vi "Start Asynchronus Logger.vi"(8 "error in (no error)":errorcluster, 10 "Queue in":refnum<queue>, 11 "Data Cluster OUT in":T1 {"Measurement Configuration"."Relative To" items=["Power sequence start", "Previous source start", "Previous source end"]; "Measurement Configuration"."Power line frequency" items=["50 Hz", "60 Hz"]; "Measurement Configuration"."Start Value" format="%#_6p"; "Measurement Configuration"."Transient Response" items=["Slow", "Normal", "Fast"]; "Measurement Configuration"."Sense Mode" items=["Local Sense", "Remote Sense"]; "Measurement Configuration"."Target Value" format="%#_6p"; "Measurement Configuration"."Source Mode" items=["DC Voltage", "DC Current"]; "Measurement Configuration"."Start Delay" format="%#_6p"; "Measurement Configuration"."Compliance Limit" format="%#_6p"; "Measurement Configuration"."Ramp Rate" format="%#_6p"}) -> (0 "error out":errorcluster, 3 "Data Cluster OUT out":T1 {"Measurement Configuration"."Relative To" items=["Power sequence start", "Previous source start", "Previous source end"]; "Measurement Configuration"."Power line frequency" items=["50 Hz", "60 Hz"]; "Measurement Configuration"."Start Value" format="%#_6p"; "Measurement Configuration"."Transient Response" items=["Slow", "Normal", "Fast"]; "Measurement Configuration"."Sense Mode" items=["Local Sense", "Remote Sense"]; "Measurement Configuration"."Target Value" format="%#_6p"; "Measurement Configuration"."Source Mode" items=["DC Voltage", "DC Current"]; "Measurement Configuration"."Start Delay" format="%#_6p"; "Measurement Configuration"."Compliance Limit" format="%#_6p"; "Measurement Configuration"."Ramp Rate" format="%#_6p"})   [LabVIEW 2024, in "devicePowerSequencerCoreLogic.lvlib"]
doc: "Starts the Asynchronous Logger to log measure data."
uses:
  devicePowerSequencerCoreLogic.lvlib
  controls/Data Cluster.ctl
  <vilib>/Plug-In SDKs/Clients/Session Management V1/Session Reservation/Session Reservation.lvclass
  <vilib>/Plug-In SDKs/Measurements/Measure Call Context/Measure Call Context.lvclass
  Measurement Configuration.ctl
  controls/Source Mode.ctl
  controls/Sense Mode.ctl
  controls/Relative To.ctl
  controls/Transient Response.ctl
  controls/Power line frequency.ctl
  Measurement Results.ctl
  controls/Channel Name.ctl
  controls/Software Flags.ctl
  controls/Ramp Configurations.ctl
  controls/Error Info.ctl
  controls/Measurements.ctl
  controls/Voltage and Current Measurements.ctl
  controls/Log Configurations.ctl
  Device Power Sequencer.lvlib
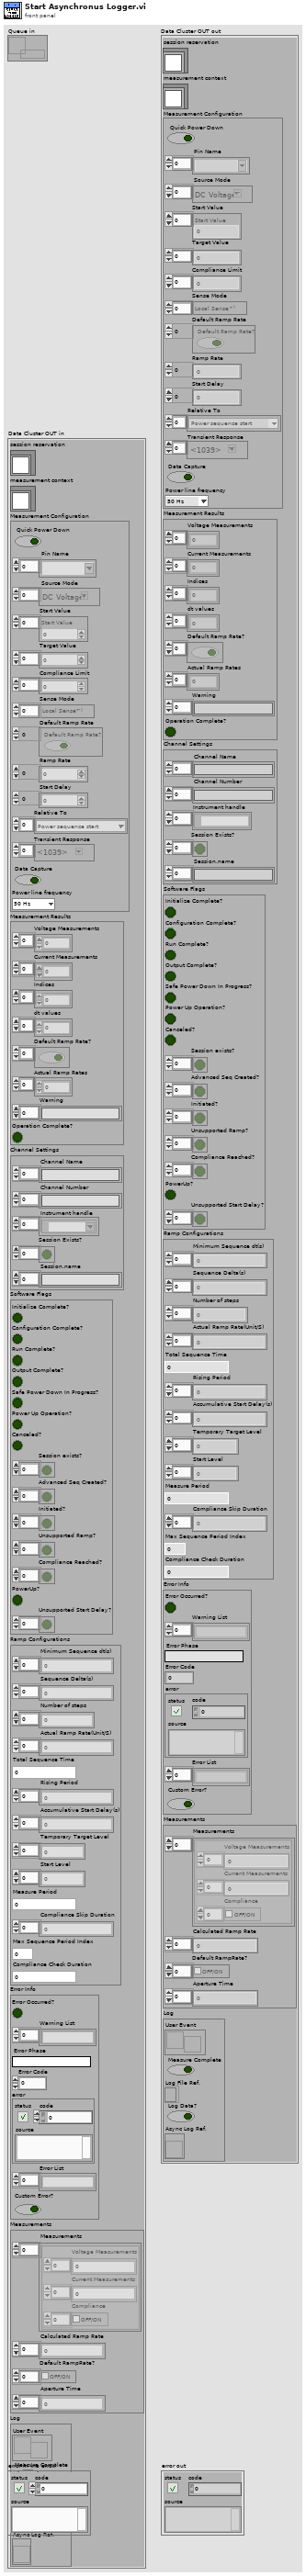
[diagram p1: front panel]
types:
  T1 = typedef "devicePowerSequencerCoreLogic.lvlib/Data Cluster.ctl" = cluster{"session reservation":refnum<class "Session Reservation.lvclass">, "measurement context":refnum<class "Measure Call Context.lvclass">, "Measurement Configuration":T2, "Measurement Results":T8, "Channel Settings":T9, "Software Flags":T10, "Ramp Configurations":T11, "Error Info":T12, "Measurements":T13, "Log":T15}
  T2 = typedef "Device Power Sequencer.lvlib/Measurement Configuration.ctl" = cluster{"Quick Power Down":bool, "Pin Name":string[], "Source Mode":T3[], "Start Value":dbl[], "Target Value":dbl[], "Compliance Limit":dbl[], "Sense Mode":T4[], "Default Ramp Rate":bool[], "Ramp Rate":dbl[], "Start Delay":dbl[], "Relative To":T5[], "Transient Response":T6[], "Data Capture":bool, "Power line frequency":T7}
  T3 = typedef "Device Power Sequencer.lvlib/Source Mode.ctl" = i32
  T4 = typedef "Device Power Sequencer.lvlib/Sense Mode.ctl" = i32
  T5 = typedef "Device Power Sequencer.lvlib/Relative To.ctl" = u32
  T6 = typedef "Device Power Sequencer.lvlib/Transient Response.ctl" = i32
  T7 = typedef "Device Power Sequencer.lvlib/Power line frequency.ctl" = u32
  T8 = typedef "Device Power Sequencer.lvlib/Measurement Results.ctl" = cluster{"Voltage Measurements":dbl[], "Current Measurements":dbl[], "Indices":i32[], "dt values":dbl[], "Default Ramp Rate?":bool[], "Actual Ramp Rates":dbl[], "Warning":string[], "Operation Complete?":bool}
  T9 = typedef "devicePowerSequencerCoreLogic.lvlib/Channel Name.ctl" = cluster{"Channel Name":string[], "Channel Number":string[], "Instrument handle":refnum<k15>[], "Session Exists?":bool[], "Session.name":string[]}
  T10 = typedef "devicePowerSequencerCoreLogic.lvlib/Software Flags.ctl" = cluster{"Initialize Complete?":bool, "Configuration Complete?":bool, "Run Complete?":bool, "Output Complete?":bool, "Safe Power Down In Progress?":bool, "Power Up Operation?":bool, "Canceled?":bool, "Session exists?":bool[], "Advanced Seq Created?":bool[], "Initiated?":bool[], "Unsupported Ramp?":bool[], "Compliance Reached?":bool[], "PowerUp?":bool, "Unsupported Start Delay?":bool[]}
  T11 = typedef "devicePowerSequencerCoreLogic.lvlib/Ramp Configurations.ctl" = cluster{"Minimum Sequence dt(s)":dbl[], "Sequence Delta(s)":dbl[], "Number of steps":i32[], "Actual Ramp Rate(Unit/S)":dbl[], "Total Sequence Time":dbl, "Rising Period":dbl[], "Accumulative Start Delay(s)":dbl[], "Temporary Target Level":dbl[], "Start Level":dbl[], "Measure Period":dbl, "Compliance Skip Duration":dbl[], "Max Sequence Period Index":i32, "Compliance Check Duration":dbl}
  T12 = typedef "devicePowerSequencerCoreLogic.lvlib/Error Info.ctl" = cluster{"Error Occurred?":bool, "Warning List":string[], "Error Phase":string, "Error Code":i32, "error":errorcluster, "Error List":string[], "Custom Error?":bool}
  T13 = typedef "devicePowerSequencerCoreLogic.lvlib/Measurements.ctl" = cluster{"Measurements":T14[], "Calculated Ramp Rate":dbl[], "Default RampRate?":bool[], "Aperture Time":dbl[]}
  T14 = typedef "devicePowerSequencerCoreLogic.lvlib/Voltage and Current Measurements.ctl" = cluster{"Voltage Measurements":dbl[], "Current Measurements":dbl[], "Compliance":bool[]}
  T15 = typedef "devicePowerSequencerCoreLogic.lvlib/Log Configurations.ctl" = cluster{"User Event":refnum<user-event>, "Measure Complete":bool, "Log File Ref.":refnum<file>, "Log Data?":bool, "Async Log Ref.":refnum<vi>}
  T16 = cluster{"Measured Data":cluster{"Voltage":dbl[], "Current":dbl[]}[], "Measure Complete":bool}
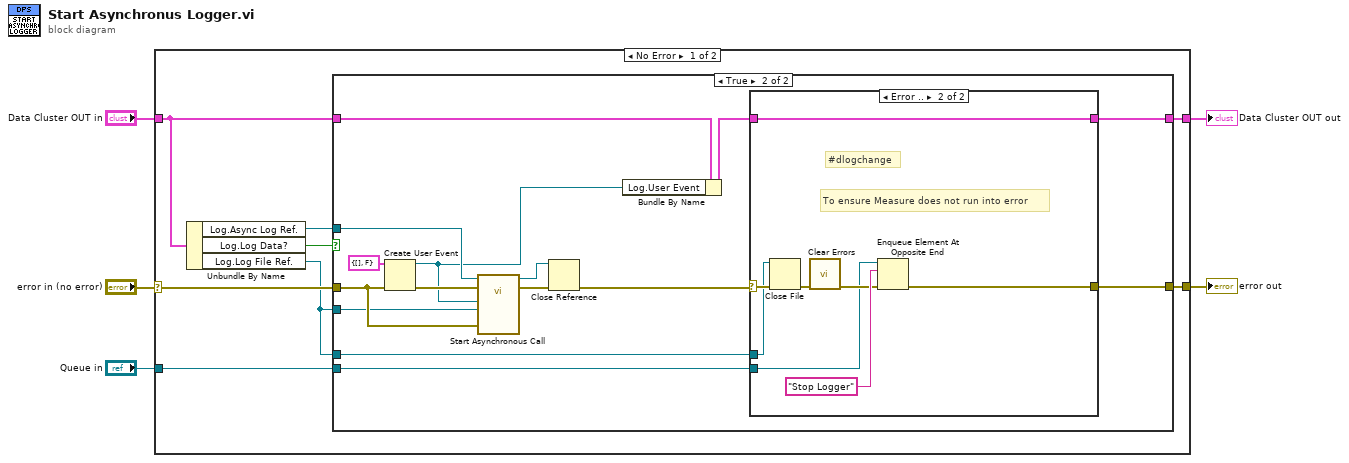
[diagram p0: block diagram]
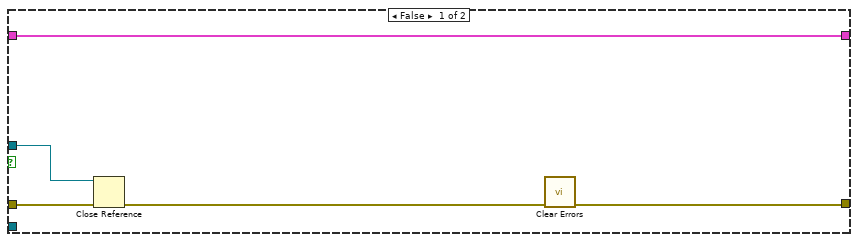
[diagram p2: hidden frame]
diagram:
  n1 = case shown="No Error" "error in (no error)" {
    selector: "error in (no error)" -> [w7 w44]
    tunnel: "Queue in" -> [w13 _]
    tunnel: "Data Cluster OUT in" -> [w12 w45]
    tunnel: [w11 w45] -> w3
    tunnel: [w8 w44] -> w2
    frame No Error {
      n2 = Unbundle By Name(w12) -> ("Log.Async Log Ref."=w10:refnum<vi>, "Log.Log Data?"=w9:bool, "Log.Log File Ref."=w6:refnum<file>)
      n3 = case shown="True" w9 {
        tunnel: [w15 w21] -> w8
        tunnel: w7 -> [w18 w29]
        tunnel: w6 -> [_ w20]
        tunnel: w10 -> [w17 w28]
        tunnel: [w16 w24] -> w11
        tunnel: w12 -> [w16 w27]
        tunnel: w13 -> [_ w23]
        tunnel: w6 -> [_ w19]
        frame False {
          n4 = Close Reference(reference=w17, error in (no error)=w18) -> (error out=w14:errorcluster)
          n5 = call <vilib>:"Clear Errors.vi"("error in (no error)"=w14) -> ("error out"=w15:errorcluster)  [unwired: 5 in, 1 out]
        }
        frame True {
          n6 = Create User Event(user event datatype=T16 {"Measured Data"=[], "Measure Complete"=FALSE} ("Measurement"), error in=w29) -> (user event=w26:refnum<user-event>, error out=w32:errorcluster)
          n7 = call-by-ref "Start Asynchronous Call"(reference=w28, error in=w32, 8:"error in (no error)"=w29, "Log File Ref."=w20, "User Event In"=w26) -> (reference out=w30:refnum<vi>, error out=w31:errorcluster)  [unwired: 8 in, 1 out]
          n8 = Close Reference(reference=w30, error in (no error)=w31) -> (error out=w22:errorcluster)
          n9 = Bundle By Name(cluster=w27, "Log.User Event"=w26) -> (w25:T1)
          n10 = case shown="Error .." w22 {
            selector: w22 -> [w35 w42]
            tunnel: [w34 w43] -> w24
            tunnel: w25 -> [w34 w43]
            tunnel: [w35 w39] -> w21
            tunnel: w23 -> [_ w38]
            tunnel: w19 -> [_ w36]
            frame No Error {
            }
            frame Error {
              # "To ensure Measure does not run into error"
              # "#dlogchange"
              n11 = Close File(refnum=w36, error in=w42) -> (error out=w37:errorcluster)  [unwired: 1 out]
              n12 = call <vilib>:"Clear Errors.vi"("error in (no error)"=w37) -> ("error out"=w40:errorcluster)  [unwired: 5 in, 1 out]
              n13 = Enqueue Element At Opposite End(queue=w38, element="Stop Logger", error in (no error)=w40) -> (error out=w39:errorcluster)  [unwired: 1 in, 2 out]
            }
          }
        }
      }
    }
    frame Error {
    }
  }
  "Data Cluster OUT out" <- w3
  "error out" <- w2
